vi "piezo2GeneratePositions.vi"(1 "M":i32) -> (0 "positions (z)":dbl[](array[numeric]))   [LabVIEW 2017]
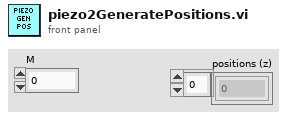
[diagram p1: front panel]
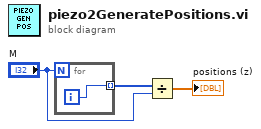
[diagram p0: block diagram]
diagram:
  n1 = for {
    N: "M" -> [_]
    tunnel: [w4] -> w3 mode=indexing
    i -> [w4]
  }
  n2 = Divide(x=w3, y="M") -> (x/y=→"positions (z)":dbl[])
